vi "KnownColor.vi"(11 "Known Color":T1(ring)=enum."DarkCyan") -> (3 "FromKnownColor":refnum<k24>)   [LabVIEW 2014, in "XMSChart.xctl"]
uses:
  XMSChart.xctl
  System.Drawing
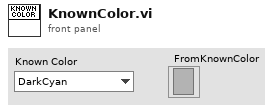
[diagram p1: front panel]
types:
  T1 = enum16{"ActiveBorder", "ActiveCaption", "ActiveCaptionText", "AppWorkspace", "Control", "ControlDark", "ControlDarkDark", "ControlLight", "ControlLightLight", "ControlText", "Desktop", "GrayText", "Highlight", "HighlightText", "HotTrack", "InactiveBorder", "InactiveCaption", "InactiveCaptionText", "Info", "InfoText", "Menu", "MenuText", "ScrollBar", "Window", "WindowFrame", "WindowText", "Transparent", "AliceBlue", "AntiqueWhite", "Aqua", "Aquamarine", "Azure", "Beige", "Bisque", "Black", "BlanchedAlmond", "Blue", "BlueViolet", "Brown", "BurlyWood", "CadetBlue", "Chartreuse", "Chocolate", "Coral", "CornflowerBlue", "Cornsilk", "Crimson", "Cyan", "DarkBlue", "DarkCyan", "DarkGoldenrod", "DarkGray", "DarkGreen", "DarkKhaki", "DarkMagenta", "DarkOliveGreen", "DarkOrange", "DarkOrchid", "DarkRed", "DarkSalmon", "DarkSeaGreen", "DarkSlateBlue", "DarkSlateGray", "DarkTurquoise", "DarkViolet", "DeepPink", "DeepSkyBlue", "DimGray", "DodgerBlue", "Firebrick", "FloralWhite", "ForestGreen", "Fuchsia", "Gainsboro", "GhostWhite", "Gold", "Goldenrod", "Gray", "Green", "GreenYellow", "Honeydew", "HotPink", "IndianRed", "Indigo", "Ivory", "Khaki", "Lavender", "LavenderBlush", "LawnGreen", "LemonChiffon", "LightBlue", "LightCoral", "LightCyan", "LightGoldenrodYellow", "LightGray", "LightGreen", "LightPink", "LightSalmon", "LightSeaGreen", "LightSkyBlue", "LightSlateGray", "LightSteelBlue", "LightYellow", "Lime", "LimeGreen", "Linen", "Magenta", "Maroon", "MediumAquamarine", "MediumBlue", "MediumOrchid", "MediumPurple", "MediumSeaGreen", "MediumSlateBlue", "MediumSpringGreen", "MediumTurquoise", "MediumVioletRed", "MidnightBlue", "MintCream", "MistyRose", "Moccasin", "NavajoWhite", "Navy", "OldLace", "Olive", "OliveDrab", "Orange", "OrangeRed", "Orchid", "PaleGoldenrod", "PaleGreen", "PaleTurquoise", "PaleVioletRed", "PapayaWhip", "PeachPuff", "Peru", "Pink", "Plum", "PowderBlue", "Purple", "Red", "RosyBrown", "RoyalBlue", "SaddleBrown", "Salmon", "SandyBrown", "SeaGreen", "SeaShell", "Sienna", "Silver", "SkyBlue", "SlateBlue", "SlateGray", "Snow", "SpringGreen", "SteelBlue", "Tan", "Teal", "Thistle", "Tomato", "Turquoise", "Violet", "Wheat", "White", "WhiteSmoke", "Yellow", "YellowGreen", "ButtonFace", "ButtonHighlight", "ButtonShadow", "GradientActiveCaption", "GradientInactiveCaption", "MenuBar", "MenuHighlight"}
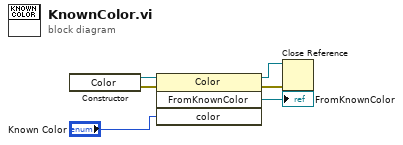
[diagram p0: block diagram]
diagram:
  n1 = constructor class="Color" ("Constructor Node")() -> (reference out=w5:refnum<k24>, error out=w6:errorcluster)  [unwired: 3 in, 1 out]
  n2 = invoke on="Invoke Node" class="Color" method="FromKnownColor"(reference=w5, error in=w6, "color"="Known Color") -> (reference out=w1:refnum<k24>, error out=w2:errorcluster, "FromKnownColor"=→"FromKnownColor":refnum<k24>)  [unwired: 1 in, 1 out]
  n3 = Close Reference(reference=w1, error in (no error)=w2) -> ()  [unwired: 1 out]
